vi "_Get Offset.vi"(5 "Index Array":i64[][](array[numeric]), 6 "Expt# (0-based)":i32=1, 7 "Scan# (1-based)":i32=1) -> (1 "Offset":i64, 3 "Scan# out":i32=1)   [LabVIEW 2012]
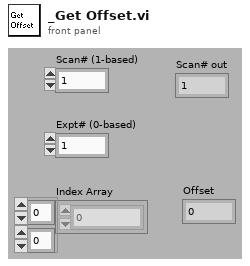
[diagram p1: front panel]
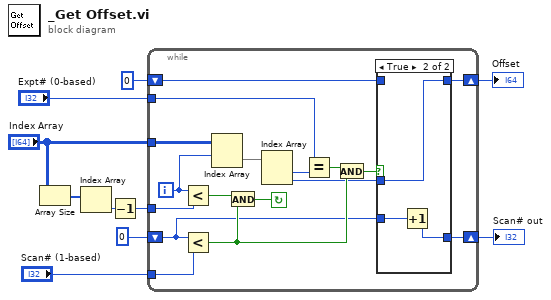
[diagram p0: block diagram]
diagram:
  n1 = Array Size(array="Index Array") -> (size(s)=w9:i32[])
  n2 = Index Array(array=w9) -> (element=w8:i32)  [unwired: 1 in]
  n3 = Decrement(x=w8) -> (x-1=w7:i32)
  n4 = while {
    tunnel: "Index Array" -> [w26]
    tunnel: w7 -> [w27]
    shift-right: [w13] -> w4
    shift-left: 0 ("Scan# (1-based)") -> [w15]
    tunnel: "Scan# (1-based)" -> [w23]
    tunnel: "Expt# (0-based)" -> [w19]
    shift-right: [w11] -> w1
    shift-left: i64 0 ("Offset") -> [w12]
    i -> [w25]
    stop <- w22 continue-if-true
    n5 = Less?(x=w25, y=w27) -> (x < y?=w24:bool)
    n6 = Less?(x=w15, y=w23) -> (x < y?=w17:bool)
    n7 = Index Array(array=w26, index (row)=w25) -> (element=w21:i64[])  [unwired: 1 in]
    n8 = And(x=w24, y=w17) -> (x .and. y?=w22:bool)
    n9 = Index Array(array=w21) -> (element #1=w20:i64, element #2=w14:i64)  [unwired: 2 in]
    n10 = Equal?(x=w19, y=w20) -> (x = y?=w18:bool)
    n11 = And(x=w18, y=w17) -> (x .and. y?=w16:bool)
    n12 = case shown="True" w16 {
      tunnel: w15 -> [w29 w32]
      tunnel: w14 -> [_ w30]
      tunnel: [w29 w31] -> w13
      tunnel: w12 -> [w28 _]
      tunnel: [w28 w30] -> w11
      frame False {
      }
      frame True {
        n13 = Increment(x=w32) -> (x+1=w31:i32)
      }
    }
  }
  "Scan# out" <- w4
  "Offset" <- w1
